vi "AlternatingLEDs.vi"() -> ()   [LabVIEW 2015]
panel:
  out "LED B":bool
  out "LED A":bool
  in  "Stop LED Pulse":bool
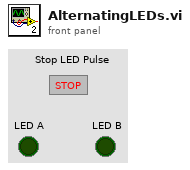
[diagram p1: front panel]
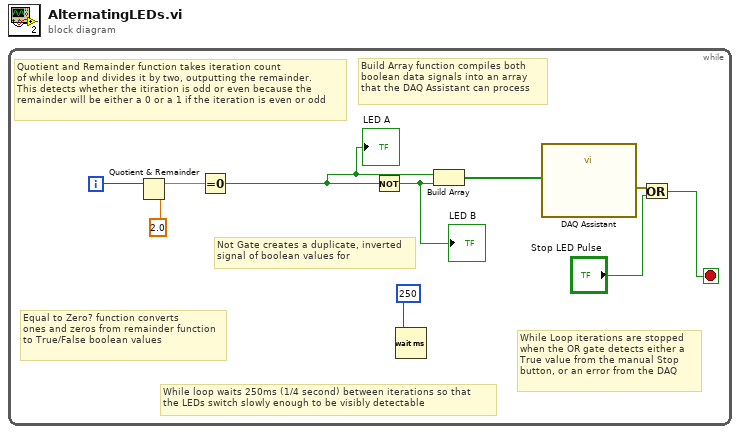
[diagram p0: block diagram]
diagram:
  n1 = while {
    i -> [w10]
    stop <- w1 stop-if-true
    # "Build Array function compiles both\nboolean data signals into an array\nthat the DAQ Assistant can process"
    # "Not Gate creates a duplicate, inverted\nsignal of boolean values for"
    # "Equal to Zero? function converts\nones and zeros from remainder function to True/False boolean values"
    # "Quotient and Remainder function takes iteration count \nof while loop and divides it by two, outputting the remainder.\nThis detects whether the itiration is odd or even because the\nremainder will be either a 0 or a 1 if the iteration is even or odd"
    # "While loop waits 250ms (1/4 second) between iterations so that\nthe LEDs switch slowly enough to be visibly detectable"
    # "While Loop iterations are stopped\nwhen the OR gate detects either a \nTrue value from the manual Stop \nbutton, or an error from the DAQ"
    n2 = Quotient & Remainder(x=w10, y=2.0 ("floor(x/y)")) -> (x-y*floor(x/y)=w8:dbl)  [unwired: 1 out]
    n3 = Equal To 0?(x=w8) -> (x = 0?=w2:bool)
    "LED A" <- w2
    n4 = Not(x=w2) -> (.not. x?=w3:bool)
    "LED B" <- w3
    n5 = Wait (ms)(milliseconds to wait=250) -> ()  [unwired: 1 out]
    n6 = Build Array(w2, w3) -> (w7:bool[])
    n7 = call "DAQ Assistant"("data"=w7) -> ("error out"=w5:errorcluster)  [unwired: 17 in, 1 out]
    n8 = Or(x=w5, y="Stop LED Pulse") -> (x .or. y?=w1:bool)
  }
